vi "SubtractCircuralBuffer.vi"(8 "BufferLength":u16=8000, 10 "y":i32, 11 "x":i32) -> (3 "z":i32)   [LabVIEW 2020]
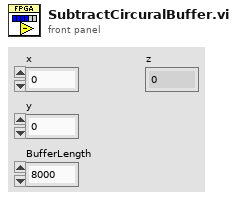
[diagram p1: front panel]
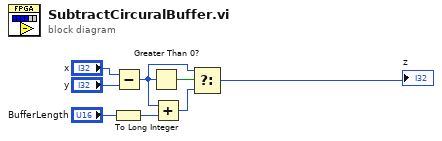
[diagram p0: block diagram]
diagram:
  n1 = To Long Integer(number="BufferLength") -> (32bit integer=w1:i32)
  n2 = Subtract(x="x", y="y") -> (x-y=w3:i32)
  n3 = Greater Than 0?(x=w3) -> (x > 0?=w2:bool)
  n4 = Add(x=w3, y=w1) -> (x+y=w5:i32)
  n5 = Select(t=w3, s=w2, f=w5) -> (s? t:f=→"z":i32)
